vi "CLD 7 Time Stamp to String Challenge Exercise.vi"(8 "Error In":errorcluster) -> (0 "Error Out":errorcluster, 3 "Code String Out":string)   [LabVIEW 2020]
doc: "CLD 7 exercise"
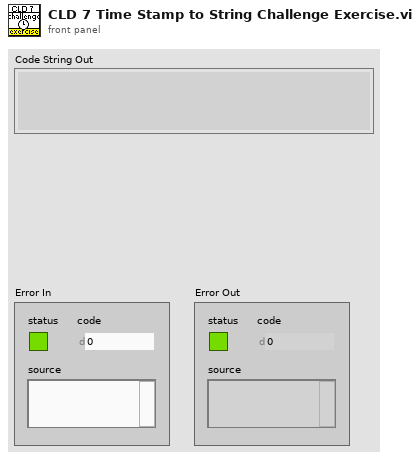
[diagram p1: front panel]
types:
  T1 = typedef "LVDateTimeRec.ctl" = cluster{"fractional second":dbl, "second":i32, "minute":i32, "hour":i32, "day of month":i32, "month":i32, "year":i32, "day of week":i32, "day of year":i32, "DST":i32}
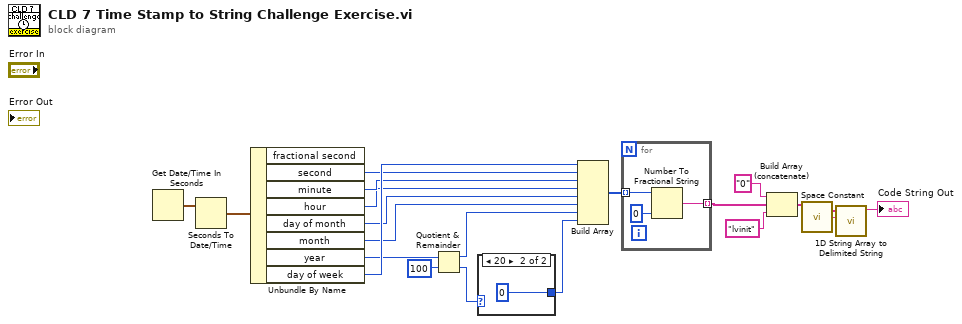
[diagram p0: block diagram]
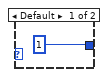
[diagram p2: hidden frame]
diagram:
  n1 = Get Date/Time In Seconds() -> (seconds since 1Jan1904=w20:timestamp)
  n2 = Seconds To Date/Time(time stamp (now)=w20) -> (date time rec=w19:T1)  [unwired: 1 in]
  n3 = Unbundle By Name(w19) -> ("second"=w15:i32, "minute"=w14:i32, "hour"=w13:i32, "day of month"=w12:i32, "month"=w11:i32, "year"=w8:i32, "day of week"=w16:i32)  [unwired: 1 out]
  n4 = Quotient & Remainder(x=w8, y=100) -> (x-y*floor(x/y)=w9:i32, floor(x/y)=w7:i32)
  n5 = case shown="20" w7 {
    tunnel: [1 0] -> w6
    frame Default {
    }
    frame 20 {
    }
  }
  n6 = Build Array(w16, w15, w14, w13, w12, w11, w9, w6) -> (w5:i32[])
  n7 = for {
    tunnel: w5 -> [w25] mode=indexing
    tunnel: [w24] -> w4 mode=indexing
    n8 = Number To Fractional String(number=w25, precision (6)=i16 0) -> (F-format string=w24:string)  [unwired: 2 in]
  }
  n9 = Build Array (concatenate)("0" ("string"), w4, "lvinit" ("string")) -> (w1:string[])
  n10 = call <vilib>:"Space Constant.vi"() -> ("String"=w18:string)
  n11 = call <vilib>:"1D String Array to Delimited String.vi"("delimiter"=w18, "string array"=w1) -> ("delimited string"=→"Code String Out":string)  [unwired: 9 in]
